vi "Periodic Tasks.vi"(8 "error in":errorcluster) -> ()   [LabVIEW 2020]
doc: "This VI runs in parallel to other tasks. It can contain as many user-defined periodic loops as you need. These can carry out PID or other sorts of timed response."
uses:
  <vilib>/Rock Robotics/WPI/DriverStation/WPI_DriverStationRobotMode2.ctl
  <vilib>/Rock Robotics/WPI/ThirdParty/Phoenix-LabVIEW/Motor Controller/Controls/CTRE_Phoenix_MotorControl_ControlMode.ctl
  <vilib>/Rock Robotics/WPI/Utilities/WPI_GetSetVariantRefNum.vi
  <vilib>/Rock Robotics/Network Tables/NT Write Numeric Array.vi
  Robot Global Data.vi
  <vilib>/Rock Robotics/Network Tables/NT Write Boolean Array.vi
  <vilib>/Rock Robotics/Network Tables/NT Write Boolean.vi
  <vilib>/Rock Robotics/WPI/RobotDrive/WPI_RobotDriveMecanumDrive_Cartesian.vi
  <vilib>/Rock Robotics/WPI/ThirdParty/Phoenix-LabVIEW/Motor Controller/Get/CTRE_Phoenix_MotorController_GetQuadratureData.vi
  <vilib>/Rock Robotics/Network Tables/NT Write Number.vi
panel:
  out "Grabber Motor Intake 2":bool
  out "Grabber Motor Outtake 2":bool
  out "Grabber Motor Outtake":bool
  out "Grabber Motor Intake":bool
  out "EncoderTR":dbl
  out "HallEffectLow":bool=TRUE
  out "HallEffectHigh":bool=TRUE
  out "EncoderER":dbl
  out "EncoderEL":dbl
  out "Slow Speed ON":bool
  out "Backwards ON":bool
  # "s"
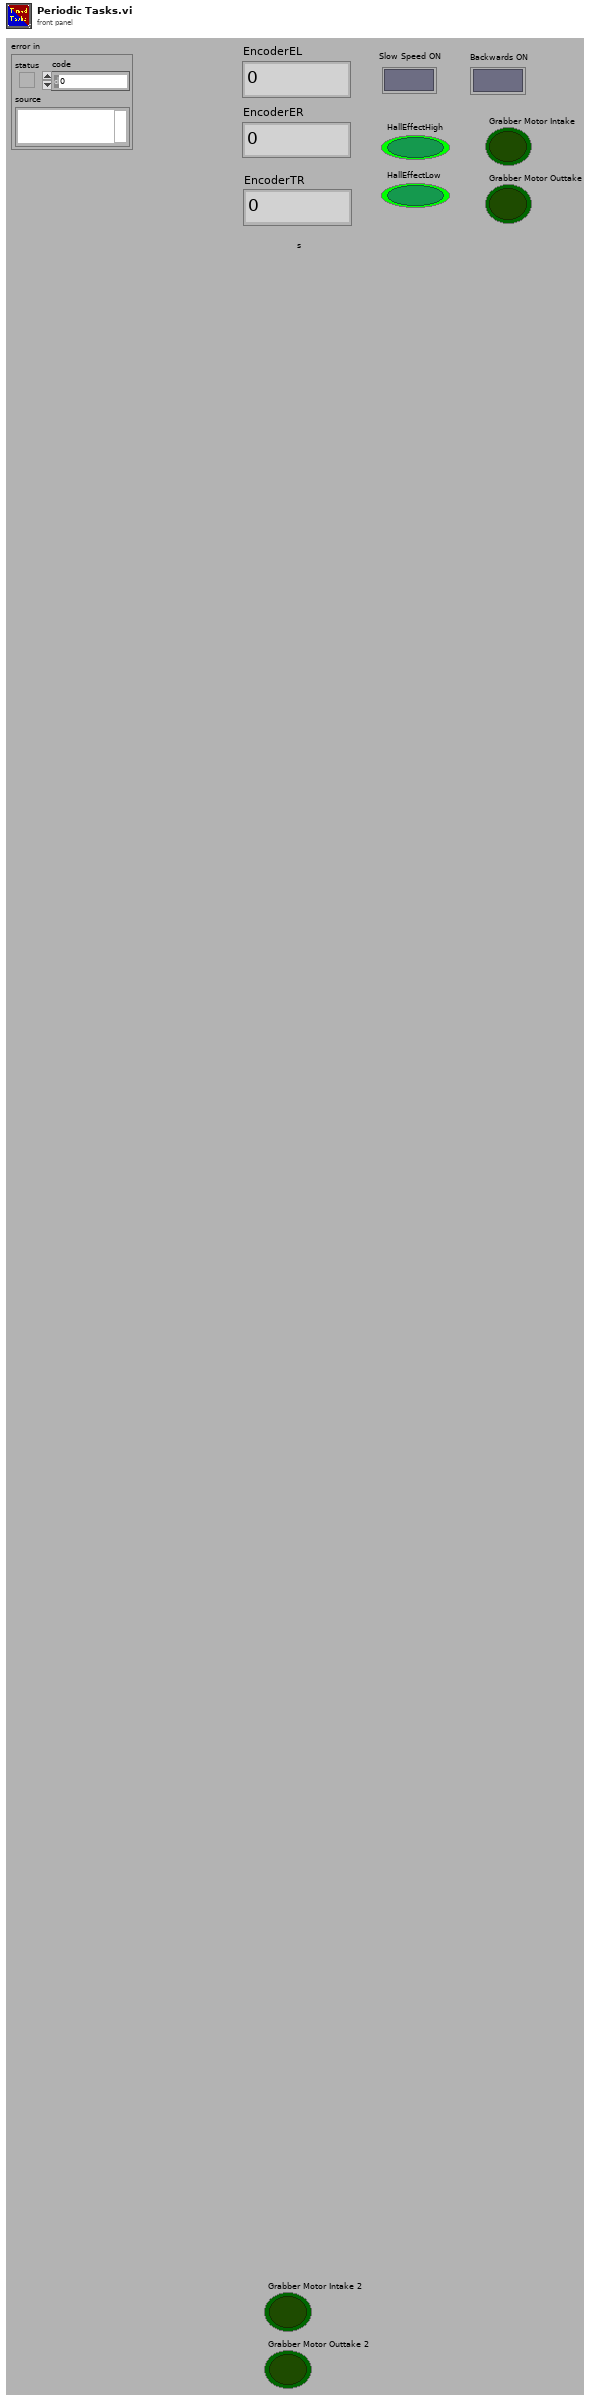
[diagram p1: front panel]
types:
  T1 = typedef "WPI_MotorControlDeviceRef.ctl" = cluster{"DeviceStatus":errorcluster, "Type":T2, "PWM":cluster{"PWM Channel":T3, "DeadBand":T4}, "CAN":cluster{"Device Number":u8, "SetOutput VI Ref":variant, "GetOutput VI Ref":variant, "Enable VI Ref":variant, "Disable VI Ref":variant, "Data":variant}, "Invert":bool, "DIO PWM":cluster{"PWM \"Enable\" Channel":T3, "DIOChannel":T5, "PWM Rate":dbl}}
  T2 = typedef "WPI_MotorControlType.ctl" = enum16{"PWM", "CAN", "DIO PWM"}
  T3 = typedef "FPGA_DIOPWMChannel.ctl" = enum8{"PWM 0", "PWM 1", "PWM 2", "PWM 3", "PWM 4", "PWM 5", "PWM 6", "PWM 7", "PWM 8", "PWM 9", "PWM MXP 0", "PWM MXP 1", "PWM MXP 2", "PWM MXP 3", "PWM MXP 4", "PWM MXP 5", "PWM MXP 6", "PWM MXP 7", "PWM MXP 8", "PWM MXP 9", "Invalid"}
  T4 = typedef "WPI_PWMDeadband.ctl" = cluster{"Name":string, "maxPositivePwm":i32, "minPositivePwm":i32, "centerPwm":i32, "maxNegativePwm":i32, "minNegativePwm":i32, "angularRange":u16}
  T5 = typedef "FPGA_DIOChannel.ctl" = enum8{"DIO 0", "DIO 1", "DIO 2", "DIO 3", "DIO 4", "DIO 5", "DIO 6", "DIO 7", "DIO 8", "DIO 9", "DIO MXP 0", "DIO MXP 1", "DIO MXP 2", "DIO MXP 3", "DIO MXP 4", "DIO MXP 5", "DIO MXP 6", "DIO MXP 7", "DIO MXP 8", "DIO MXP 9", "DIO MXP 10", "DIO MXP 11", "DIO MXP 12", "DIO MXP 13", "DIO MXP 14", "DIO MXP 15", "SPI Port CS1", "SPI Port CS2", "SPI Port CS3", "SPI Port MISO", "SPI Port MOSI", "Invalid"}
  T6 = typedef "WPI_JoystickDevRef.ctl" = cluster{"Device":T7}
  T7 = typedef "WPI_JoystickDeviceEnum.ctl" = enum16{"USB 0", "USB 1", "USB 2", "USB 3", "USB 4", "USB 5"}
  T8 = typedef "WPI_RobotDriveDevRef.ctl" = cluster{"DevStatus":errorcluster, "Motors[]":T1[], "Square Inputs":bool, "Max Output":dbl}
  T9 = typedef "WPI_DigitalInputDevRef.ctl" = cluster{"DevStatus":errorcluster, "DIO Channel":T5}
  T10 = typedef "WPI_DriverStationRobotMode2.ctl" = enum16{"Autonomous Disabled", "Autonomous Enabled", "Teleop Disabled", "Teleop Enabled", "Disconnected", "Finish", "Test Disabled", "Test Enabled", "Emergency Stopped"}
  T11 = enum16{"DownBypass", "UpBypass", "Score", "Down", "Up", "Off"}
  T12 = typedef "CTRE_Phoenix_MotorControl_ControlMode.ctl" = u16
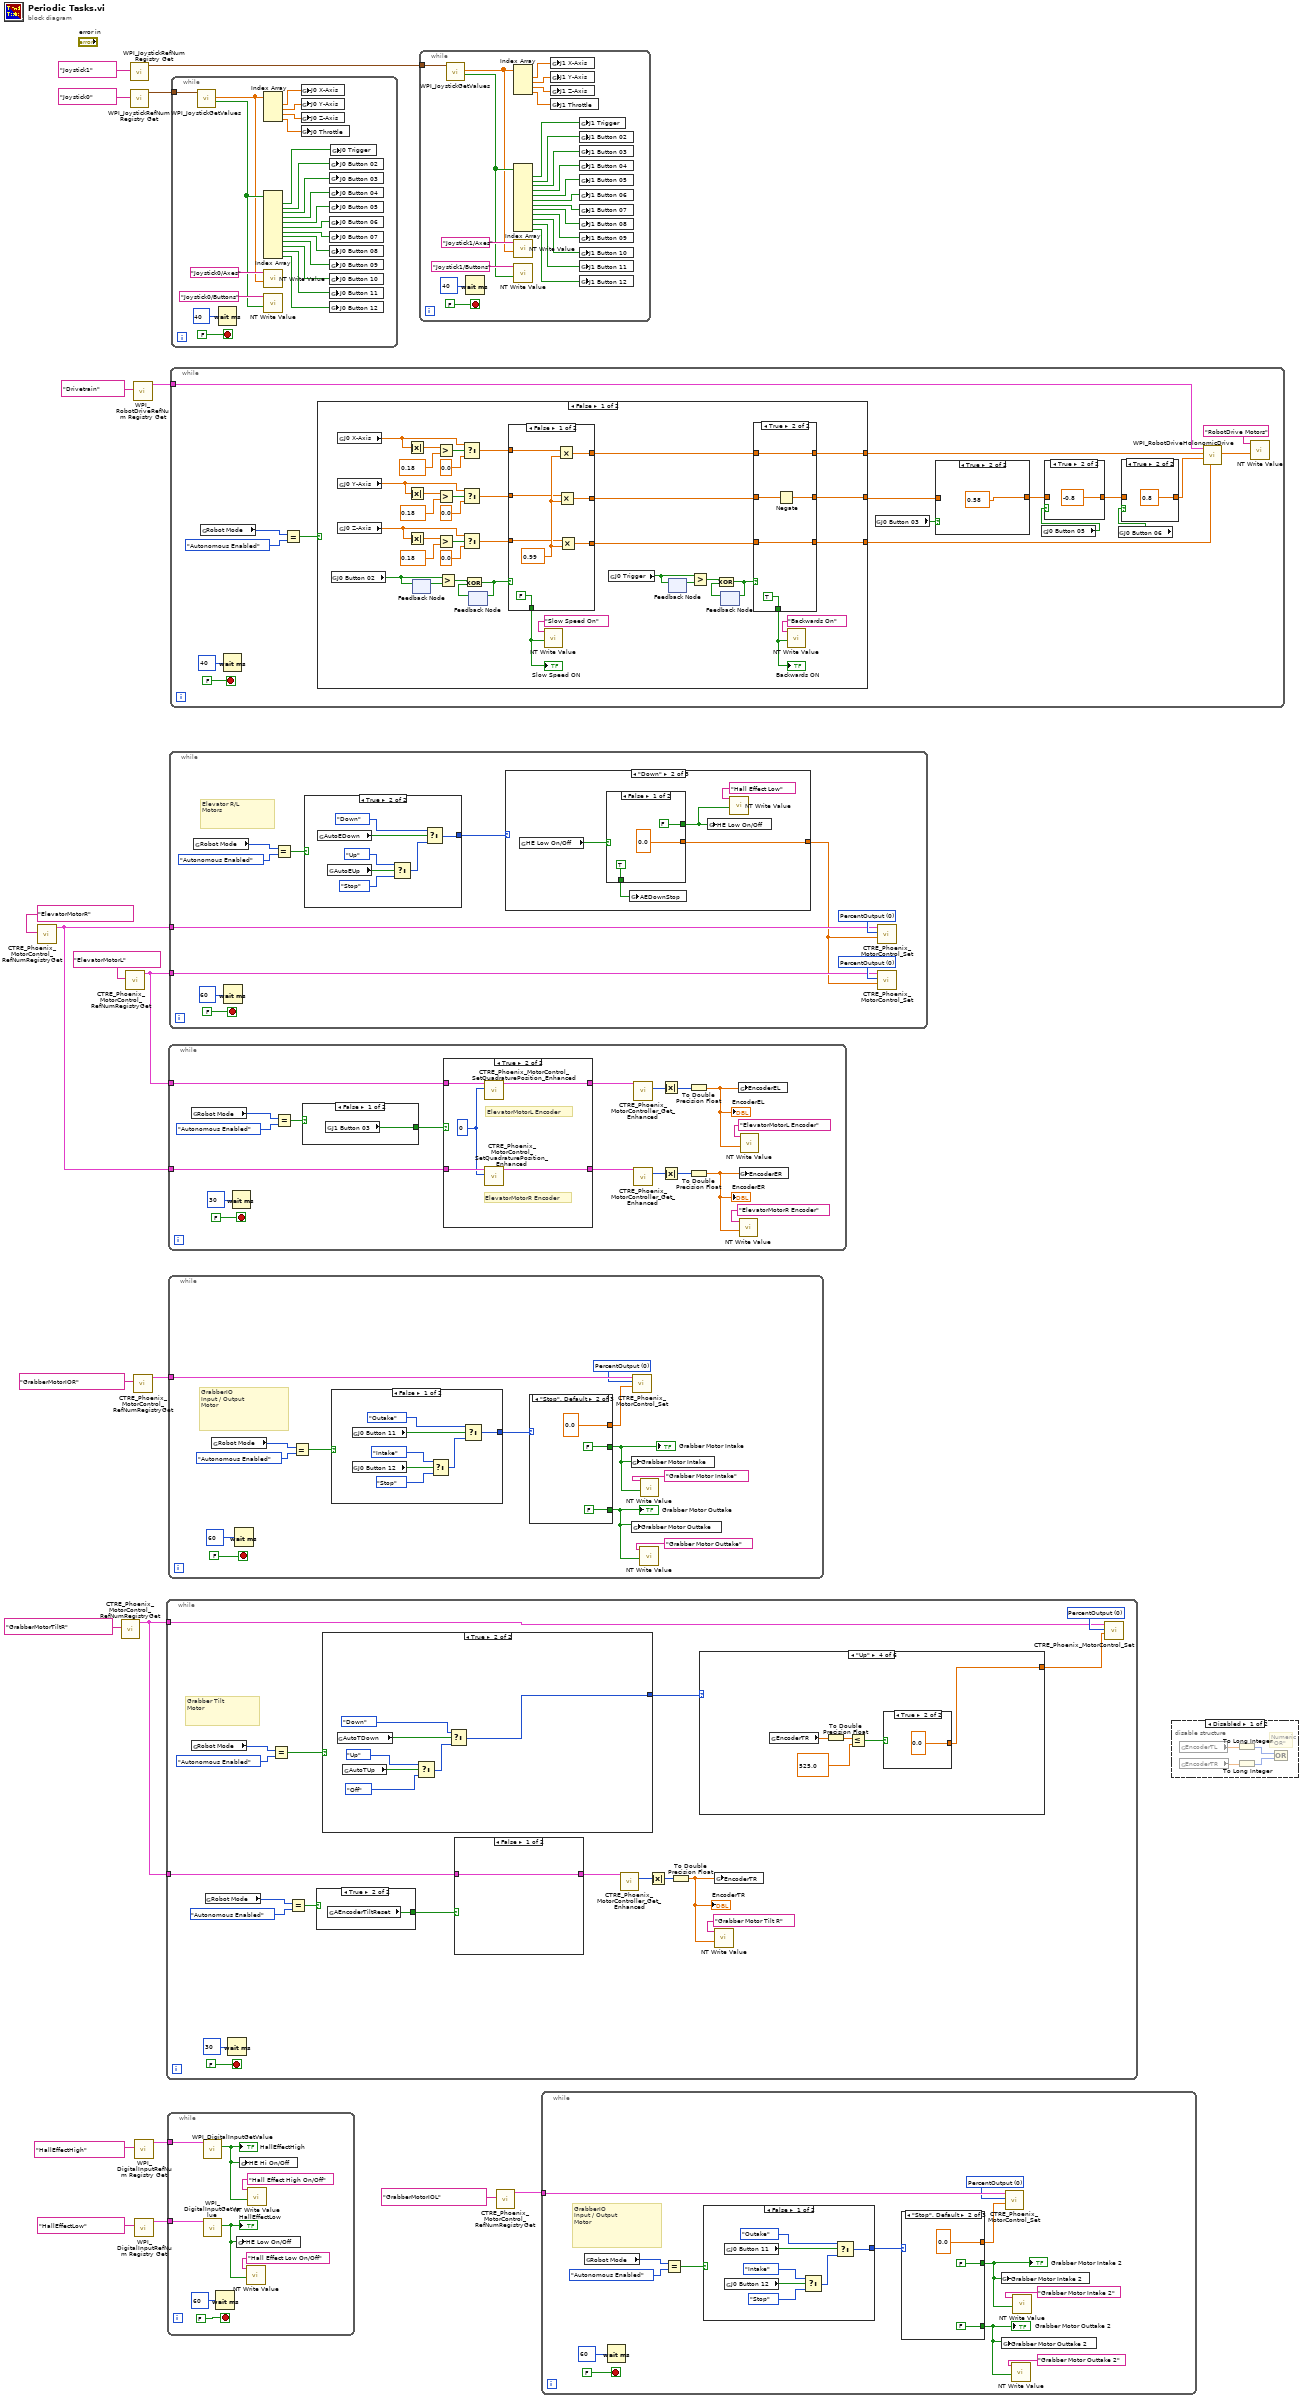
[diagram p0: block diagram]
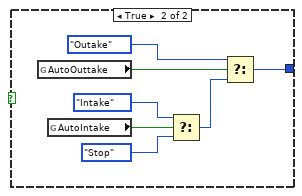
[diagram p2: hidden frame]
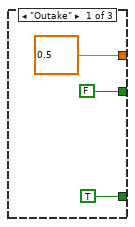
[diagram p3: hidden frame]
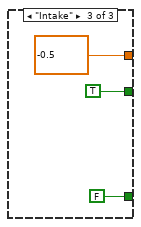
[diagram p4: hidden frame]
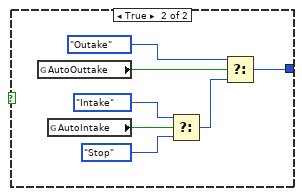
[diagram p6: hidden frame]
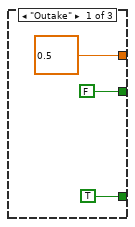
[diagram p7: hidden frame]
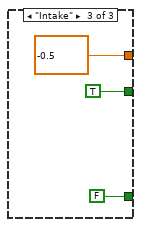
[diagram p8: hidden frame]
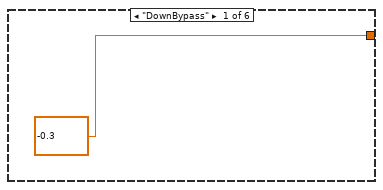
[diagram p9: hidden frame]
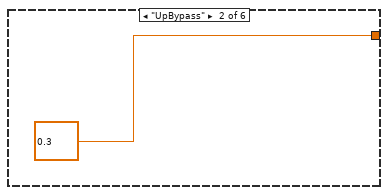
[diagram p10: hidden frame]
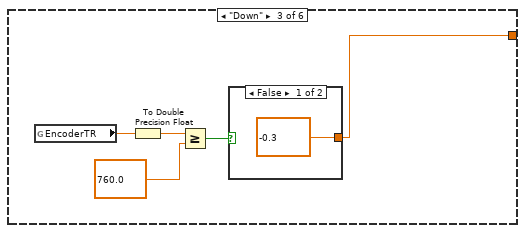
[diagram p11: hidden frame]
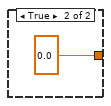
[diagram p12: hidden frame]
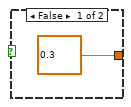
[diagram p13: hidden frame]
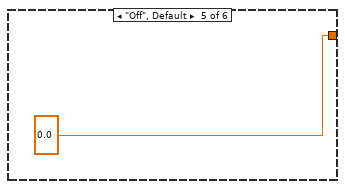
[diagram p14: hidden frame]
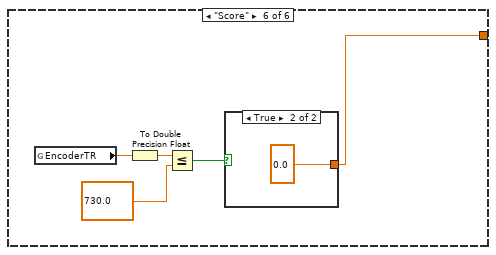
[diagram p15: hidden frame]
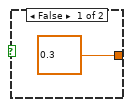
[diagram p16: hidden frame]
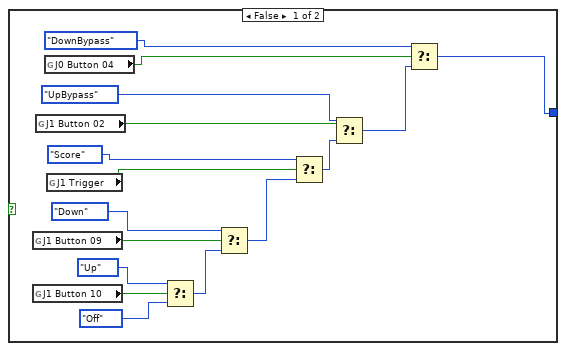
[diagram p17: hidden frame]
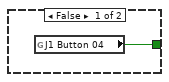
[diagram p18: hidden frame]
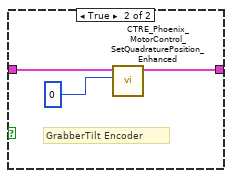
[diagram p19: hidden frame]
diagram:
  n1 = call <vilib>:"CTRE_Phoenix_MotorControl_RefNumRegistryGet.vi"("refnum name"="ElevatorMotorR") -> ("PhoenixMotorControlDevRef"=w10:T1)  [unwired: 9 in, 1 out]
  n2 = call <vilib>:"CTRE_Phoenix_MotorControl_RefNumRegistryGet.vi"("refnum name"="GrabberMotorTiltR") -> ("PhoenixMotorControlDevRef"=w4:T1)  [unwired: 9 in, 1 out]
  n3 = call <vilib>:"CTRE_Phoenix_MotorControl_RefNumRegistryGet.vi"("refnum name"="ElevatorMotorL") -> ("PhoenixMotorControlDevRef"=w11:T1)  [unwired: 9 in, 1 out]
  n4 = call <vilib>:"WPI_JoystickRefNum Registry Get.vi"("refnum name"="Joystick1") -> ("JoystickDevRef"=w16:T6)  [unwired: 1 in, 9 out]
  n5 = call <vilib>:"WPI_JoystickRefNum Registry Get.vi"("refnum name"="Joystick0") -> ("JoystickDevRef"=w18:T6)  [unwired: 1 in, 9 out]
  n6 = call <vilib>:"WPI_RobotDriveRefNum Registry Get.vi"("refnum name"="Drivetrain") -> ("RobotDriveDevRef"=w15:T8)  [unwired: 1 in, 9 out]
  n7 = call <vilib>:"CTRE_Phoenix_MotorControl_RefNumRegistryGet.vi"("refnum name"="GrabberMotorIOR") -> ("PhoenixMotorControlDevRef"=w3:T1)  [unwired: 9 in, 1 out]
  n8 = call <vilib>:"WPI_DigitalInputRefNum Registry Get.vi"("refnum name"="HallEffectHigh") -> ("DigitalInputDevRef"=w8:T9)  [unwired: 9 in, 1 out]
  n9 = call <vilib>:"WPI_DigitalInputRefNum Registry Get.vi"("refnum name"="HallEffectLow") -> ("DigitalInputDevRef"=w7:T9)  [unwired: 9 in, 1 out]
  n10 = while {
    tunnel: w4 -> [w38]
    tunnel: w4 -> [w33]
    stop <- FALSE stop-if-true
    w39 = T12 0 items=["PercentOutput"=0, "Position"=1, "Velocity"=2, "Current"=3, "Follower"=5, "MotionProfile"=6, "MotionMagic"=7, "MotionProfileArc"=10, "Disabled"=15] ("Control Mode")
    # "Grabber Tilt\nMotor"
    n11 = global read "Robot Global Data.vi" "Robot Mode"() -> (w25:T10)
    n12 = global read "Robot Global Data.vi" "Robot Mode"() -> (w32:T10)
    n13 = Wait (ms)(milliseconds to wait=u32 30) -> ()  [unwired: 1 out]
    n14 = Equal?(x=w25, y=WPI_DriverStationRobotMode2."Autonomous Enabled") -> (x = y?=w23:bool)
    n15 = Equal?(x=w32, y=WPI_DriverStationRobotMode2."Autonomous Enabled") -> (x = y?=w30:bool)
    n16 = case shown="True" w30 {
      tunnel: [w87 w88] -> w28
      frame False {
        n17 = global read "Robot Global Data.vi" "J1 Button 04"() -> (w87:bool)
      }
      frame True {
        n18 = global read "Robot Global Data.vi" "AEncoderTiltReset"() -> (w88:bool)
      }
    }
    n19 = case shown="True" w23 {
      tunnel: [w64 w83] -> w22
      frame False {
        n20 = global read "Robot Global Data.vi" "J1 Button 09"() -> (w78:bool)
        n21 = global read "Robot Global Data.vi" "J1 Button 10"() -> (w77:bool)
        n22 = global read "Robot Global Data.vi" "J1 Button 02"() -> (w73:bool)
        n23 = global read "Robot Global Data.vi" "J0 Button 04"() -> (w66:bool)
        n24 = global read "Robot Global Data.vi" "J1 Trigger"() -> (w75:bool)
        n25 = Select(t=T11."Up", s=w77, f=T11."Off") -> (s? t:f=w79:T11)
        n26 = Select(t=T11."Down", s=w78, f=w79) -> (s? t:f=w74:T11)
        n27 = Select(t=T11."Score", s=w75, f=w74) -> (s? t:f=w72:T11)
        n28 = Select(t=T11."UpBypass", s=w73, f=w72) -> (s? t:f=w65:T11)
        n29 = Select(t=T11."DownBypass", s=w66, f=w65) -> (s? t:f=w64:T11)
      }
      frame True {
        n30 = global read "Robot Global Data.vi" "AutoTDown"() -> (w85:bool)
        n31 = global read "Robot Global Data.vi" "AutoTUp"() -> (w84:bool)
        n32 = Select(t=T11."Up", s=w84, f=T11."Off") -> (s? t:f=w86:T11)
        n33 = Select(t=T11."Down", s=w85, f=w86) -> (s? t:f=w83:T11)
      }
    }
    n34 = case shown="False" w28 {
      tunnel: w33 -> [w89 w92]
      tunnel: [w89 w91] -> w29
      frame False {
      }
      frame True {
        # "GrabberTilt Encoder"
        n35 = call <vilib>:"CTRE_Phoenix_MotorControl_SetQuadraturePosition_Enhanced.vi"("New Position"=0, "PhoenixMotorControlDevRef"=w92) -> ("PhoenixMotorControlDevRef"=w91:T1)  [unwired: 8 in, 1 out]
      }
    }
    n36 = call-poly <vilib>:"CTRE_Phoenix_MotorController_Get_Enhanced.vi"("PhoenixMotorControlDevRef"=w29) -> ("Quadrature Position"=w37:i32)  [unwired: 11 in, 3 out]
    n37 = Absolute Value(x=w37) -> (abs(x)=w36:i32)
    n38 = To Double Precision Float(number=w36) -> (double precision float=w34:dbl)
    "EncoderTR" <- w34
    n39 = case shown="\"Up\"" w22 {
      tunnel: [-0.3 0.3 w42 w49 0.0 w57] -> w21
      frame "DownBypass" {
      }
      frame "UpBypass" {
      }
      frame "Down" {
        n40 = global read "Robot Global Data.vi" "EncoderTR"() -> (w46:dbl)
        n41 = To Double Precision Float(number=w46) -> (double precision float=w44:dbl)
        n42 = Greater Or Equal?(x=w44, y=760.0) -> (x >= y?=w45:bool)
        n43 = case shown="False" w45 {
          tunnel: [-0.3 0.0] -> w42
          frame False {
          }
          frame True {
          }
        }
      }
      frame "Up" {
        n44 = global read "Robot Global Data.vi" "EncoderTR"() -> (w51:dbl)
        n45 = To Double Precision Float(number=w51) -> (double precision float=w53:dbl)
        n46 = Less Or Equal?(x=w53, y=525.0) -> (x <= y?=w52:bool)
        n47 = case shown="True" w52 {
          tunnel: [0.3 0.0] -> w49
          frame False {
          }
          frame True {
          }
        }
      }
      frame "Off", Default {
      }
      frame "Score" {
        n48 = global read "Robot Global Data.vi" "EncoderTR"() -> (w59:dbl)
        n49 = To Double Precision Float(number=w59) -> (double precision float=w61:dbl)
        n50 = Less Or Equal?(x=w61, y=730.0) -> (x <= y?=w60:bool)
        n51 = case shown="True" w60 {
          tunnel: [0.3 0.0] -> w57
          frame False {
          }
          frame True {
          }
        }
      }
    }
    n52 = global write "Robot Global Data.vi" "EncoderTR"(w34) -> ()
    n53 = call-poly <vilib>:"NT Write Value.vi"("Numeric"=w34, "Name"="Grabber Motor Tilt R") -> ()  [unwired: 9 in, 1 out]
    n54 = call <vilib>:"CTRE_Phoenix_MotorControl_Set.vi"("Output"=w21, "Control Mode"=w39, "PhoenixMotorControlDevRef"=w38) -> ()  [unwired: 7 in, 2 out]
  }
  n55 = while {
    tunnel: w8 -> [w98]
    tunnel: w7 -> [w97]
    stop <- FALSE stop-if-true
    n56 = call <vilib>:"WPI_DigitalInputGetValue.vi"("DigitalInputDevRef"=w98) -> ("Value"=w94:bool)  [unwired: 8 in, 2 out]
    "HallEffectHigh" <- w94
    n57 = call <vilib>:"WPI_DigitalInputGetValue.vi"("DigitalInputDevRef"=w97) -> ("Value"=w93:bool)  [unwired: 8 in, 2 out]
    "HallEffectLow" <- w93
    n58 = Wait (ms)(milliseconds to wait=u32 60) -> ()  [unwired: 1 out]
    n59 = global write "Robot Global Data.vi" "HE Low On/Off"(w93) -> ()
    n60 = global write "Robot Global Data.vi" "HE Hi On/Off"(w94) -> ()
    n61 = call-poly <vilib>:"NT Write Value.vi"("Boolean"=w93, "Name"="Hall Effect Low On/Off") -> ()  [unwired: 9 in, 1 out]
    n62 = call-poly <vilib>:"NT Write Value.vi"("Boolean"=w94, "Name"="Hall Effect High On/Off") -> ()  [unwired: 9 in, 1 out]
  }
  n63 = while {
    tunnel: w11 -> [w115]
    tunnel: w10 -> [w114]
    stop <- FALSE stop-if-true
    n64 = global read "Robot Global Data.vi" "Robot Mode"() -> (w118:T10)
    n65 = Wait (ms)(milliseconds to wait=u32 30) -> ()  [unwired: 1 out]
    n66 = Equal?(x=w118, y=WPI_DriverStationRobotMode2."Autonomous Enabled") -> (x = y?=w116:bool)
    n67 = case shown="False" w116 {
      tunnel: [w126 w127] -> w113
      frame False {
        n68 = global read "Robot Global Data.vi" "J1 Button 03"() -> (w126:bool)
      }
      frame True {
        n69 = global read "Robot Global Data.vi" "AEncoderElevatorReset"() -> (w127:bool)
      }
    }
    n70 = case shown="True" w113 {
      tunnel: w115 -> [w120 w125]
      tunnel: w114 -> [w119 w124]
      tunnel: [w120 w123] -> w112
      tunnel: [w119 w122] -> w111
      frame False {
      }
      frame True {
        w121 = 0
        # "ElevatorMotorL Encoder"
        # "ElevatorMotorR Encoder"
        n71 = call <vilib>:"CTRE_Phoenix_MotorControl_SetQuadraturePosition_Enhanced.vi"("New Position"=w121, "PhoenixMotorControlDevRef"=w125) -> ("PhoenixMotorControlDevRef"=w123:T1)  [unwired: 8 in, 1 out]
        n72 = call <vilib>:"CTRE_Phoenix_MotorControl_SetQuadraturePosition_Enhanced.vi"("New Position"=w121, "PhoenixMotorControlDevRef"=w124) -> ("PhoenixMotorControlDevRef"=w122:T1)  [unwired: 8 in, 1 out]
      }
    }
    n73 = call-poly <vilib>:"CTRE_Phoenix_MotorController_Get_Enhanced.vi"("PhoenixMotorControlDevRef"=w112) -> ("Quadrature Position"=w110:i32)  [unwired: 11 in, 3 out]
    n74 = call-poly <vilib>:"CTRE_Phoenix_MotorController_Get_Enhanced.vi"("PhoenixMotorControlDevRef"=w111) -> ("Quadrature Position"=w109:i32)  [unwired: 11 in, 3 out]
    n75 = Absolute Value(x=w110) -> (abs(x)=w107:i32)
    n76 = Absolute Value(x=w109) -> (abs(x)=w108:i32)
    n77 = To Double Precision Float(number=w107) -> (double precision float=w101:dbl)
    "EncoderEL" <- w101
    n78 = To Double Precision Float(number=w108) -> (double precision float=w102:dbl)
    "EncoderER" <- w102
    n79 = global write "Robot Global Data.vi" "EncoderEL"(w101) -> ()
    n80 = global write "Robot Global Data.vi" "EncoderER"(w102) -> ()
    n81 = call-poly <vilib>:"NT Write Value.vi"("Numeric"=w102, "Name"="ElevatorMotorR Encoder") -> ()  [unwired: 9 in, 1 out]
    n82 = call-poly <vilib>:"NT Write Value.vi"("Numeric"=w101, "Name"="ElevatorMotorL Encoder") -> ()  [unwired: 9 in, 1 out]
  }
  n83 = while {
    tunnel: w3 -> [w137]
    stop <- FALSE stop-if-true
    w132 = T12 0 items=["PercentOutput"=0, "Position"=1, "Velocity"=2, "Current"=3, "Follower"=5, "MotionProfile"=6, "MotionMagic"=7, "MotionProfileArc"=10, "Disabled"=15] ("Control Mode")
    # "GrabberIO\nInput / Output\nMotor"
    n84 = global read "Robot Global Data.vi" "Robot Mode"() -> (w136:T10)
    n85 = Wait (ms)(milliseconds to wait=u32 60) -> ()  [unwired: 1 out]
    n86 = Equal?(x=w136, y=WPI_DriverStationRobotMode2."Autonomous Enabled") -> (x = y?=w134:bool)
    n87 = case shown="False" w134 {
      tunnel: [w141 w148] -> w133
      frame False {
        n88 = global read "Robot Global Data.vi" "J0 Button 11"() -> (w143:bool)
        n89 = global read "Robot Global Data.vi" "J0 Button 12"() -> (w145:bool)
        n90 = Select(t=enum16{"Outake", "Intake", "Stop"}."Intake", s=w145, f=enum16{"Outake", "Intake", "Stop"}."Stop") -> (s? t:f=w142:enum16{"Outake", "Intake", "Stop"})
        n91 = Select(t=enum16{"Outake", "Intake", "Stop"}."Outake", s=w143, f=w142) -> (s? t:f=w141:enum16{"Outake", "Intake", "Stop"})
      }
      frame True {
        n92 = global read "Robot Global Data.vi" "AutoOuttake"() -> (w150:bool)
        n93 = global read "Robot Global Data.vi" "AutoIntake"() -> (w152:bool)
        n94 = Select(t=enum16{"Outake", "Intake", "Stop"}."Intake", s=w152, f=enum16{"Outake", "Intake", "Stop"}."Stop") -> (s? t:f=w149:enum16{"Outake", "Intake", "Stop"})
        n95 = Select(t=enum16{"Outake", "Intake", "Stop"}."Outake", s=w150, f=w149) -> (s? t:f=w148:enum16{"Outake", "Intake", "Stop"})
      }
    }
    n96 = case shown="\"Stop\", Default" w133 {
      tunnel: [0.5 0.0 -0.5] -> w138
      tunnel: [FALSE FALSE TRUE] -> w128
      tunnel: [TRUE FALSE FALSE] -> w129
      frame "Outake" {
      }
      frame "Stop", Default {
      }
      frame "Intake" {
      }
    }
    "Grabber Motor Intake" <- w128
    "Grabber Motor Outtake" <- w129
    n97 = global write "Robot Global Data.vi" "Grabber Motor Intake"(w128) -> ()
    n98 = global write "Robot Global Data.vi" "Grabber Motor Outtake"(w129) -> ()
    n99 = call <vilib>:"CTRE_Phoenix_MotorControl_Set.vi"("Output"=w138, "Control Mode"=w132, "PhoenixMotorControlDevRef"=w137) -> ()  [unwired: 7 in, 2 out]
    n100 = call-poly <vilib>:"NT Write Value.vi"("Boolean"=w129, "Name"="Grabber Motor Outtake") -> ()  [unwired: 9 in, 1 out]
    n101 = call-poly <vilib>:"NT Write Value.vi"("Boolean"=w128, "Name"="Grabber Motor Intake") -> ()  [unwired: 9 in, 1 out]
  }
  n102 = while {
    tunnel: w10 -> [w166]
    tunnel: w11 -> [w168]
    stop <- FALSE stop-if-true
    w169 = T12 0 items=["PercentOutput"=0, "Position"=1, "Velocity"=2, "Current"=3, "Follower"=5, "MotionProfile"=6, "MotionMagic"=7, "MotionProfileArc"=10, "Disabled"=15] ("Control Mode")
    w167 = T12 0 items=["PercentOutput"=0, "Position"=1, "Velocity"=2, "Current"=3, "Follower"=5, "MotionProfile"=6, "MotionMagic"=7, "MotionProfileArc"=10, "Disabled"=15] ("Control Mode")
    # "Elevator R/L\nMotors"
    n103 = global read "Robot Global Data.vi" "Robot Mode"() -> (w172:T10)
    n104 = Wait (ms)(milliseconds to wait=u32 60) -> ()  [unwired: 1 out]
    n105 = Equal?(x=w172, y=WPI_DriverStationRobotMode2."Autonomous Enabled") -> (x = y?=w170:bool)
    n106 = case shown="True" w170 {
      tunnel: [w198 w205] -> w164
      frame False {
        n107 = global read "Robot Global Data.vi" "J1 Button 11"() -> (w203:bool)
        n108 = global read "Robot Global Data.vi" "J1 Button 12"() -> (w204:bool)
        n109 = Select(t=enum16{"Up", "Down", "Stop"}."Up", s=w204, f=enum16{"Up", "Down", "Stop"}."Stop") -> (s? t:f=w202:enum16{"Up", "Down", "Stop"})
        n110 = Select(t=enum16{"Up", "Down", "Stop"}."Down", s=w203, f=w202) -> (s? t:f=w198:enum16{"Up", "Down", "Stop"})
      }
      frame True {
        n111 = global read "Robot Global Data.vi" "AutoEDown"() -> (w209:bool)
        n112 = global read "Robot Global Data.vi" "AutoEUp"() -> (w210:bool)
        n113 = Select(t=enum16{"Up", "Down", "Stop"}."Up", s=w210, f=enum16{"Up", "Down", "Stop"}."Stop") -> (s? t:f=w211:enum16{"Up", "Down", "Stop"})
        n114 = Select(t=enum16{"Up", "Down", "Stop"}."Down", s=w209, f=w211) -> (s? t:f=w205:enum16{"Up", "Down", "Stop"})
      }
    }
    n115 = case shown="\"Down\"" w164 {
      tunnel: [w179 w190 0.0] -> w165
      frame "Up" {
        n116 = global read "Robot Global Data.vi" "HE Hi On/Off"() -> (w177:bool)
        n117 = case shown="False" w177 {
          tunnel: [TRUE ("AUpStop") FALSE ("AUpStop")] -> w176
          tunnel: [FALSE ("AUpStop") TRUE ("AUpStop")] -> w175
          tunnel: [0.0 0.4] -> w179
          frame False {
          }
          frame True {
          }
        }
        n118 = global write "Robot Global Data.vi" "AEUpStop"(w176) -> ()
        n119 = global write "Robot Global Data.vi" "HE Hi On/Off"(w175) -> ()
        n120 = call-poly <vilib>:"NT Write Value.vi"("Boolean"=w175, "Name"="Hall Effect High") -> ()  [unwired: 9 in, 1 out]
      }
      frame "Down" {
        n121 = global read "Robot Global Data.vi" "HE Low On/Off"() -> (w188:bool)
        n122 = case shown="False" w188 {
          tunnel: [TRUE ("ADownStop") FALSE ("ADownStop")] -> w189
          tunnel: [FALSE ("ADownStop") TRUE ("ADownStop")] -> w187
          tunnel: [0.0 -0.4] -> w190
          frame False {
          }
          frame True {
          }
        }
        n123 = global write "Robot Global Data.vi" "AEDownStop"(w189) -> ()
        n124 = global write "Robot Global Data.vi" "HE Low On/Off"(w187) -> ()
        n125 = call-poly <vilib>:"NT Write Value.vi"("Boolean"=w187, "Name"="Hall Effect Low") -> ()  [unwired: 9 in, 1 out]
      }
      frame "Stop", Default {
      }
    }
    n126 = call <vilib>:"CTRE_Phoenix_MotorControl_Set.vi"("Output"=w165, "Control Mode"=w167, "PhoenixMotorControlDevRef"=w166) -> ()  [unwired: 7 in, 2 out]
    n127 = call <vilib>:"CTRE_Phoenix_MotorControl_Set.vi"("Output"=w165, "Control Mode"=w169, "PhoenixMotorControlDevRef"=w168) -> ()  [unwired: 7 in, 2 out]
  }
  n128 = while {
    tunnel: w15 -> [w222]
    stop <- FALSE stop-if-true
    n129 = global read "Robot Global Data.vi" "Robot Mode"() -> (w227:T10)
    n130 = Wait (ms)(milliseconds to wait=u32 40) -> ()  [unwired: 1 out]
    n131 = Equal?(x=w227, y=WPI_DriverStationRobotMode2."Autonomous Enabled") -> (x = y?=w225:bool)
    n132 = case shown="False" w225 {
      tunnel: [w237 w299] -> w219
      tunnel: [w236 w298] -> w218
      tunnel: [w235 w300] -> w220
      frame False {
        n133 = global read "Robot Global Data.vi" "J0 Button 02"() -> (w247:bool)
        n134 = global read "Robot Global Data.vi" "J0 X-Axis"() -> (w251:dbl)
        n135 = global read "Robot Global Data.vi" "J0 Y-Axis"() -> (w250:dbl)
        n136 = global read "Robot Global Data.vi" "J0 Z-Axis"() -> (w249:dbl)
        n137 = Absolute Value(x=w251) -> (abs(x)=w266:dbl)
        n138 = Absolute Value(x=w250) -> (abs(x)=w268:dbl)
        n139 = Absolute Value(x=w249) -> (abs(x)=w260:dbl)
        n140 = feedback #1() -> (w271:bool)  [unwired: 1 in]
        n141 = feedback-in #1(w247) -> ()
        n142 = Greater?(x=w266, y=0.18) -> (0:w267:bool)
        n143 = Greater?(x=w268, y=0.18) -> (0:w269:bool)
        n144 = Greater?(x=w260, y=0.18) -> (0:w261:bool)
        n145 = Greater?(x=w247, y=w271) -> (0:w270:bool)
        n146 = Select(t=w251, s=w267, f=0.0) -> (s? t:f=w252:dbl)
        n147 = Select(t=w250, s=w269, f=0.0) -> (s? t:f=w253:dbl)
        n148 = Select(t=w249, s=w261, f=0.0) -> (s? t:f=w254:dbl)
        n149 = feedback #2() -> (w272:bool)  [unwired: 1 in]
        n150 = Exclusive Or(1:w272, 2:w270) -> (0:w248:bool)
        n151 = feedback-in #2(w248) -> ()
        n152 = case shown="False" w248 {
          tunnel: w252 -> [w288 w297]
          tunnel: w253 -> [w287 w296]
          tunnel: [w285 w295] -> w240
          tunnel: [w284 w294] -> w239
          tunnel: w254 -> [w286 w292]
          tunnel: [w283 w291] -> w238
          tunnel: [FALSE ("Boolean") TRUE ("Boolean")] -> w246
          frame False {
            w289 = 0.99 ("y")
            n153 = Multiply(x=w288, y=w289) -> (x*y=w285:dbl)
            n154 = Multiply(x=w287, y=w289) -> (x*y=w284:dbl)
            n155 = Multiply(x=w286, y=w289) -> (x*y=w283:dbl)
          }
          frame True {
            w293 = 0.6 ("y")
            n156 = Multiply(x=w297, y=w293) -> (x*y=w295:dbl)
            n157 = Multiply(x=w296, y=w293) -> (x*y=w294:dbl)
            n158 = Multiply(x=w292, y=w293) -> (x*y=w291:dbl)
          }
        }
        "Slow Speed ON" <- w246
        n159 = call-poly <vilib>:"NT Write Value.vi"("Boolean"=w246, "Name"="Slow Speed On") -> ()  [unwired: 9 in, 1 out]
        n160 = global read "Robot Global Data.vi" "J0 Trigger"() -> (w245:bool)
        n161 = feedback #3() -> (w244:bool)  [unwired: 1 in]
        n162 = feedback-in #3(w245) -> ()
        n163 = Greater?(x=w245, y=w244) -> (0:w255:bool)
        n164 = feedback #4() -> (w243:bool)  [unwired: 1 in]
        n165 = Exclusive Or(1:w243, 2:w255) -> (0:w242:bool)
        n166 = feedback-in #4(w242) -> ()
        n167 = case shown="True" w242 {
          tunnel: w239 -> [w275 w280]
          tunnel: w240 -> [w273 w278]
          tunnel: [w275 w279] -> w236
          tunnel: [w273 w278] -> w235
          tunnel: w238 -> [w274 w277]
          tunnel: [w274 w277] -> w237
          tunnel: [FALSE ("Boolean") TRUE ("Boolean")] -> w241
          frame False {
          }
          frame True {
            n168 = Negate(x=w280) -> (-x=w279:dbl)
          }
        }
        "Backwards ON" <- w241
        n169 = call-poly <vilib>:"NT Write Value.vi"("Boolean"=w241, "Name"="Backwards On") -> ()  [unwired: 9 in, 1 out]
      }
      frame True {
        n170 = global read "Robot Global Data.vi" "ADriveRotate"() -> (w299:dbl)
        n171 = global read "Robot Global Data.vi" "ADriveStrafe"() -> (w300:dbl)
        n172 = global read "Robot Global Data.vi" "ADriveFR"() -> (w298:dbl)
      }
    }
    n173 = global read "Robot Global Data.vi" "J0 Button 03"() -> (w217:bool)
    n174 = case shown="True" w217 {
      tunnel: w218 -> [w233 _]
      tunnel: [w233 0.58 ("y")] -> w214
      frame False {
      }
      frame True {
      }
    }
    n175 = global read "Robot Global Data.vi" "J0 Button 05"() -> (w215:bool)
    n176 = case shown="True" w215 {
      tunnel: w214 -> [w231 _]
      tunnel: [w231 -0.8 ("y")] -> w213
      frame False {
      }
      frame True {
      }
    }
    n177 = global read "Robot Global Data.vi" "J0 Button 06"() -> (w216:bool)
    n178 = case shown="True" w216 {
      tunnel: w213 -> [w229 _]
      tunnel: [w229 0.8 ("y")] -> w212
      frame False {
      }
      frame True {
      }
    }
    n179 = call-poly <vilib>:"WPI_RobotDriveHolonomicDrive.vi"("Rotation"=w219, "Y"=w212, "X"=w220, "RobotDriveDevRef"=w222) -> ("Motor Values"=w221:dbl[])  [unwired: 5 in, 2 out]
    n180 = call-poly <vilib>:"NT Write Value.vi"("Numeric Array"=w221, "Name"="RobotDrive Motors") -> ()  [unwired: 9 in, 1 out]
  }
  n181 = while {
    tunnel: w18 -> [w321]
    stop <- FALSE stop-if-true
    n182 = call <vilib>:"WPI_JoystickGetValues.vi"("JoystickDevRef"=w321) -> ("Buttons"=w302:bool[], "Axes"=w301:dbl[])  [unwired: 6 in, 3 out]
    n183 = Wait (ms)(milliseconds to wait=u32 40) -> ()  [unwired: 1 out]
    n184 = Index Array(array=w301) -> (element #1=w320:dbl, element #2=w319:dbl, element #3=w318:dbl, element #4=w317:dbl)  [unwired: 4 in]
    n185 = Index Array(array=w302) -> (element #1=w316:bool, element #2=w315:bool, element #3=w314:bool, element #4=w313:bool, element #5=w312:bool, element #6=w311:bool, element #7=w310:bool, element #8=w309:bool, element #9=w308:bool, element #10=w307:bool, element #11=w306:bool, element #12=w305:bool)  [unwired: 12 in]
    n186 = call-poly <vilib>:"NT Write Value.vi"("Numeric Array"=w301, "Name"="Joystick0/Axes") -> ()  [unwired: 9 in, 1 out]
    n187 = call-poly <vilib>:"NT Write Value.vi"("Boolean Array"=w302, "Name"="Joystick0/Buttons") -> ()  [unwired: 9 in, 1 out]
    n188 = global write "Robot Global Data.vi" "J0 X-Axis"(w320) -> ()
    n189 = global write "Robot Global Data.vi" "J0 Y-Axis"(w319) -> ()
    n190 = global write "Robot Global Data.vi" "J0 Z-Axis"(w318) -> ()
    n191 = global write "Robot Global Data.vi" "J0 Throttle"(w317) -> ()
    n192 = global write "Robot Global Data.vi" "J0 Button 02"(w315) -> ()
    n193 = global write "Robot Global Data.vi" "J0 Button 03"(w314) -> ()
    n194 = global write "Robot Global Data.vi" "J0 Button 04"(w313) -> ()
    n195 = global write "Robot Global Data.vi" "J0 Button 05"(w312) -> ()
    n196 = global write "Robot Global Data.vi" "J0 Button 06"(w311) -> ()
    n197 = global write "Robot Global Data.vi" "J0 Button 07"(w310) -> ()
    n198 = global write "Robot Global Data.vi" "J0 Button 08"(w309) -> ()
    n199 = global write "Robot Global Data.vi" "J0 Button 09"(w308) -> ()
    n200 = global write "Robot Global Data.vi" "J0 Button 10"(w307) -> ()
    n201 = global write "Robot Global Data.vi" "J0 Button 11"(w306) -> ()
    n202 = global write "Robot Global Data.vi" "J0 Button 12"(w305) -> ()
    n203 = global write "Robot Global Data.vi" "J0 Trigger"(w316) -> ()
  }
  n204 = while {
    tunnel: w16 -> [w344]
    stop <- FALSE stop-if-true
    n205 = call <vilib>:"WPI_JoystickGetValues.vi"("JoystickDevRef"=w344) -> ("Buttons"=w325:bool[], "Axes"=w324:dbl[])  [unwired: 6 in, 3 out]
    n206 = Wait (ms)(milliseconds to wait=u32 40) -> ()  [unwired: 1 out]
    n207 = Index Array(array=w324) -> (element #1=w343:dbl, element #2=w342:dbl, element #3=w341:dbl, element #4=w340:dbl)  [unwired: 4 in]
    n208 = Index Array(array=w325) -> (element #1=w339:bool, element #2=w338:bool, element #3=w337:bool, element #4=w336:bool, element #5=w335:bool, element #6=w334:bool, element #7=w333:bool, element #8=w332:bool, element #9=w331:bool, element #10=w330:bool, element #11=w329:bool, element #12=w328:bool)  [unwired: 12 in]
    n209 = call-poly <vilib>:"NT Write Value.vi"("Numeric Array"=w324, "Name"="Joystick1/Axes") -> ()  [unwired: 9 in, 1 out]
    n210 = call-poly <vilib>:"NT Write Value.vi"("Boolean Array"=w325, "Name"="Joystick1/Buttons") -> ()  [unwired: 9 in, 1 out]
    n211 = global write "Robot Global Data.vi" "J1 X-Axis"(w343) -> ()
    n212 = global write "Robot Global Data.vi" "J1 Y-Axis"(w342) -> ()
    n213 = global write "Robot Global Data.vi" "J1 Z-Axis"(w341) -> ()
    n214 = global write "Robot Global Data.vi" "J1 Throttle"(w340) -> ()
    n215 = global write "Robot Global Data.vi" "J1 Trigger"(w339) -> ()
    n216 = global write "Robot Global Data.vi" "J1 Button 02"(w338) -> ()
    n217 = global write "Robot Global Data.vi" "J1 Button 03"(w337) -> ()
    n218 = global write "Robot Global Data.vi" "J1 Button 04"(w336) -> ()
    n219 = global write "Robot Global Data.vi" "J1 Button 05"(w335) -> ()
    n220 = global write "Robot Global Data.vi" "J1 Button 06"(w334) -> ()
    n221 = global write "Robot Global Data.vi" "J1 Button 07"(w333) -> ()
    n222 = global write "Robot Global Data.vi" "J1 Button 08"(w332) -> ()
    n223 = global write "Robot Global Data.vi" "J1 Button 09"(w331) -> ()
    n224 = global write "Robot Global Data.vi" "J1 Button 10"(w330) -> ()
    n225 = global write "Robot Global Data.vi" "J1 Button 11"(w329) -> ()
    n226 = global write "Robot Global Data.vi" "J1 Button 12"(w328) -> ()
  }
  n227 = call <vilib>:"CTRE_Phoenix_MotorControl_RefNumRegistryGet.vi"("refnum name"="GrabberMotorIOL") -> ("PhoenixMotorControlDevRef"=w1:T1)  [unwired: 9 in, 1 out]
  n228 = while {
    tunnel: w1 -> [w356]
    stop <- FALSE stop-if-true
    w351 = T12 0 items=["PercentOutput"=0, "Position"=1, "Velocity"=2, "Current"=3, "Follower"=5, "MotionProfile"=6, "MotionMagic"=7, "MotionProfileArc"=10, "Disabled"=15] ("Control Mode")
    # "GrabberIO\nInput / Output\nMotor"
    n229 = global read "Robot Global Data.vi" "Robot Mode"() -> (w355:T10)
    n230 = Wait (ms)(milliseconds to wait=u32 60) -> ()  [unwired: 1 out]
    n231 = Equal?(x=w355, y=WPI_DriverStationRobotMode2."Autonomous Enabled") -> (x = y?=w353:bool)
    n232 = case shown="False" w353 {
      tunnel: [w360 w367] -> w352
      frame False {
        n233 = global read "Robot Global Data.vi" "J0 Button 11"() -> (w362:bool)
        n234 = global read "Robot Global Data.vi" "J0 Button 12"() -> (w364:bool)
        n235 = Select(t=enum16{"Outake", "Intake", "Stop"}."Intake", s=w364, f=enum16{"Outake", "Intake", "Stop"}."Stop") -> (s? t:f=w361:enum16{"Outake", "Intake", "Stop"})
        n236 = Select(t=enum16{"Outake", "Intake", "Stop"}."Outake", s=w362, f=w361) -> (s? t:f=w360:enum16{"Outake", "Intake", "Stop"})
      }
      frame True {
        n237 = global read "Robot Global Data.vi" "AutoOuttake"() -> (w369:bool)
        n238 = global read "Robot Global Data.vi" "AutoIntake"() -> (w371:bool)
        n239 = Select(t=enum16{"Outake", "Intake", "Stop"}."Intake", s=w371, f=enum16{"Outake", "Intake", "Stop"}."Stop") -> (s? t:f=w368:enum16{"Outake", "Intake", "Stop"})
        n240 = Select(t=enum16{"Outake", "Intake", "Stop"}."Outake", s=w369, f=w368) -> (s? t:f=w367:enum16{"Outake", "Intake", "Stop"})
      }
    }
    n241 = case shown="\"Stop\", Default" w352 {
      tunnel: [0.5 0.0 -0.5] -> w357
      tunnel: [FALSE FALSE TRUE] -> w347
      tunnel: [TRUE FALSE FALSE] -> w348
      frame "Outake" {
      }
      frame "Stop", Default {
      }
      frame "Intake" {
      }
    }
    "Grabber Motor Intake 2" <- w347
    "Grabber Motor Outtake 2" <- w348
    n242 = global write "Robot Global Data.vi" "Grabber Motor Intake 2"(w347) -> ()
    n243 = global write "Robot Global Data.vi" "Grabber Motor Outtake 2"(w348) -> ()
    n244 = call <vilib>:"CTRE_Phoenix_MotorControl_Set.vi"("Output"=w357, "Control Mode"=w351, "PhoenixMotorControlDevRef"=w356) -> ()  [unwired: 7 in, 2 out]
    n245 = call-poly <vilib>:"NT Write Value.vi"("Boolean"=w348, "Name"="Grabber Motor Outtake 2") -> ()  [unwired: 9 in, 1 out]
    n246 = call-poly <vilib>:"NT Write Value.vi"("Boolean"=w347, "Name"="Grabber Motor Intake 2") -> ()  [unwired: 9 in, 1 out]
  }
  n247 = disable-structure shown="Disabled" {
    frame Disabled {
      # "Numeric\n\"OR\""
      n248 = global read "Robot Global Data.vi" "EncoderTL"() -> (w384:dbl)
      n249 = global read "Robot Global Data.vi" "EncoderTR"() -> (w383:dbl)
      n250 = To Long Integer(number=w384) -> (32bit integer=w386:i32)
      n251 = To Long Integer(number=w383) -> (32bit integer=w385:i32)
      n252 = Compound Arithmetic op=OR(w386, w385) -> ()  [unwired: 1 out]
    }
    frame Enabled {
    }
  }
